vi "SeCrTs-AO_Scale.vi"(8 "error in (no error)":errorcluster, 10 "AO":T1(array[cluster]), 11 "Refnum in":refnum<k21>) -> (0 "error out":errorcluster, 3 "Refnum out":refnum<k21>)   [LabVIEW 2022 SP3]
uses:
  <vilib>/DAQmx/create/channels.llb/DAQmx Create Channel (AO-Voltage-Basic).vi
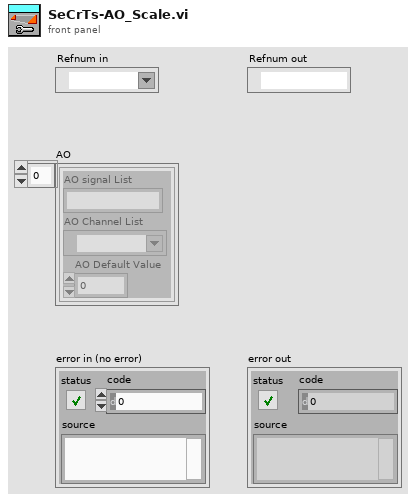
[diagram p1: front panel]
types:
  T1 = cluster{"AO signal List":string, "AO Channel List":tag, "AO Default Value":dbl}[]
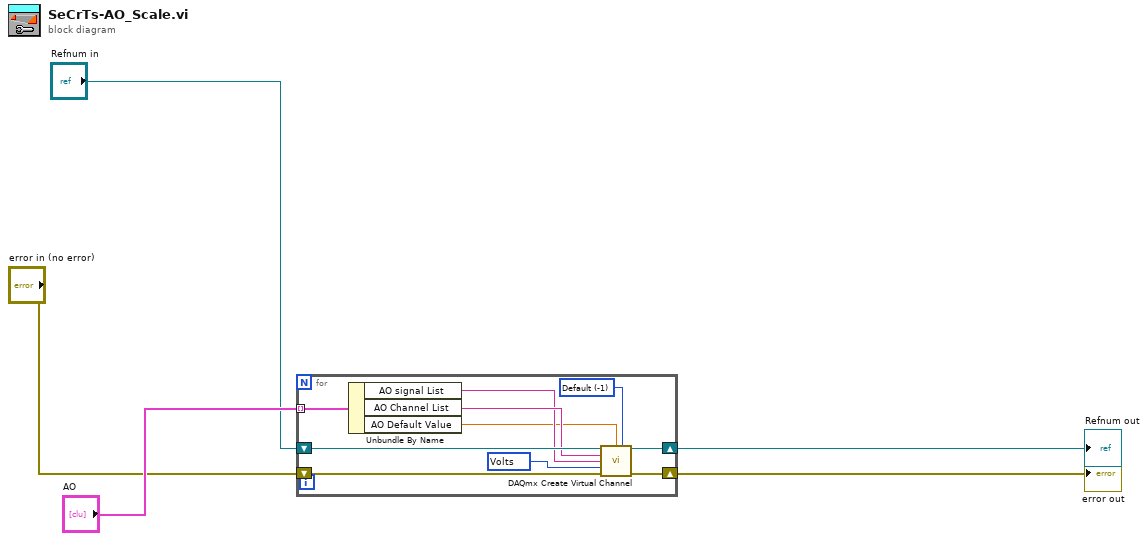
[diagram p0: block diagram]
diagram:
  n1 = for {
    shift-right: [w14] -> w1
    shift-left: "error in (no error)" -> [w8]
    tunnel: "AO" -> [w12] mode=indexing
    shift-right: [w15] -> w2
    shift-left: "Refnum in" -> [w11]
    w6 = -1 items=["Default"=-1, "RSE"=10083, "Differential"=10106, "Pseudodifferential"=12529] ("output terminal configuration")
    w13 = 10348 items=["Volts"=10348, "From Custom Scale"=10065] ("units")
    n2 = Unbundle By Name(w12) -> ("AO signal List"=w9:string, "AO Channel List"=w10:tag, "AO Default Value"=w7:dbl)
    n3 = call-poly <vilib>:"DAQmx Create Virtual Channel.vi"("task in"=w11, "minimum value"=w7, "output terminal configuration"=w6, "physical channels"=w10, "name to assign"=w9, "units"=w13, "error in"=w8) -> ("task out"=w15:refnum<k21>, "error out"=w14:errorcluster)  [unwired: 7 in]
  }
  "Refnum out" <- w2
  "error out" <- w1
